vi "Cconfigure HSDIO Pin for PPMU Voltage.vi"(8 "Error In":errorcluster, 9 "voltage level":dbl=1.8 format="%#_13g", 10 "Pins":string[](array[string])=["Vio"], 11 "Semiconductor Module Context":T1) -> (0 "Error Out":errorcluster)   [LabVIEW 2013]
uses:
  <vilib>/NI_TestStand_SemiconductorModule/NI_TestStand_Semiconductor_Module.lvlibp/PinMap/General/SemiconductorModuleContext.ctl
  <vilib>/NI_TestStand_SemiconductorModule/NI_TestStand_Semiconductor_Module.lvlibp/PinMap/General/NIInstrumentTypeIDs.ctl
  <vilib>/NI_TestStand_SemiconductorModule/NI_TestStand_Semiconductor_Module.lvlibp/PinMap/HSDIO/PinsToNIHSDIOSessions.vi
  <vilib>/NI_TestStand_SemiconductorModule/NI_TestStand_Semiconductor_Module.lvlibp
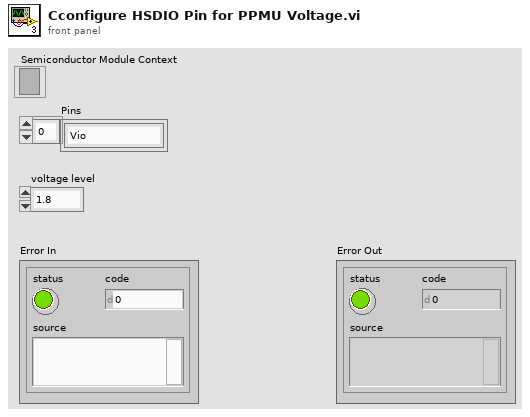
[diagram p1: front panel]
types:
  T1 = typedef "NI_TestStand_Semiconductor_Module.lvlibp/SemiconductorModuleContext.ctl" = refnum<k7>
  T2 = typedef "NI_TestStand_Semiconductor_Module.lvlibp/NIInstrumentTypeIDs.ctl" = string
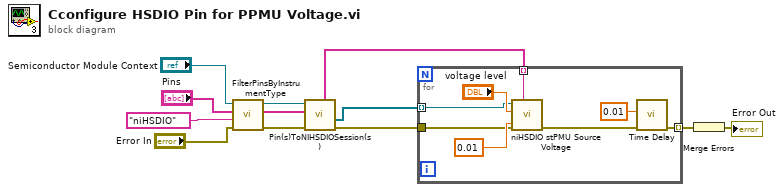
[diagram p0: block diagram]
diagram:
  n1 = call <vilib>:"FilterPinsByInstrumentType.vi"("error in (no error)"="Error In", "Instrument Type Id"=T2 "niHSDIO", "Pins"="Pins", "Semiconductor Module Context"="Semiconductor Module Context") -> ("error out"=w12:errorcluster, "Filtered Pins"=w9:string[], "Semiconductor Module Context Out"=w11:T1)  [unwired: 5 in]
  n2 = call-poly <vilib>:"Pin(s)ToNIHSDIOSession(s).vi"("error in (no error)"=w12, "Pins"=w9, "Semiconductor Module Context"=w11) -> ("error out"=w5:errorcluster, "Generation Sessions"=w7:refnum<k15>[], "Channel Lists"=w4:string[])  [unwired: 3 in, 3 out]
  n3 = for {
    tunnel: w7 -> [w18] mode=indexing
    tunnel: w5 -> [w17]
    tunnel: w4 -> [w16] mode=indexing
    tunnel: [w14] -> w2 mode=indexing
    n4 = call <instrlib>:"niHSDIO stPMU Source Voltage.vi"("current range"=0.01, "channel list"=w16, "error in (no error)"=w17, "voltage level"="voltage level", "instrument handle"=w18) -> ("error out"=w15:errorcluster)  [unwired: 5 in, 1 out]
    n5 = call "Time Delay"("error in (no error)"=w15, "Delay Time (s)"=0.01) -> ("error out"=w14:errorcluster)  [unwired: 9 out]
  }
  n6 = Merge Errors(w2) -> (→"Error Out":errorcluster)
